vi "Stop.vi"(8 "error in (no error)":errorcluster, 9 "timeout in ms (-1)":i32=-1, 11 "Process In":refnum<class "Process.lvclass">) -> (0 "error out":errorcluster, 1 "timed out?":bool, 3 "Process Out":refnum<class "Process.lvclass">)   [LabVIEW 2020, in "Process.lvclass"]
doc: "Sends a stop message to the process, which must perform a safe shut down. This VI waits for the process to call the Finish method or times out if the configured time out expires."
uses:
  Process.lvclass
  Process.lvclass/Process.ctl
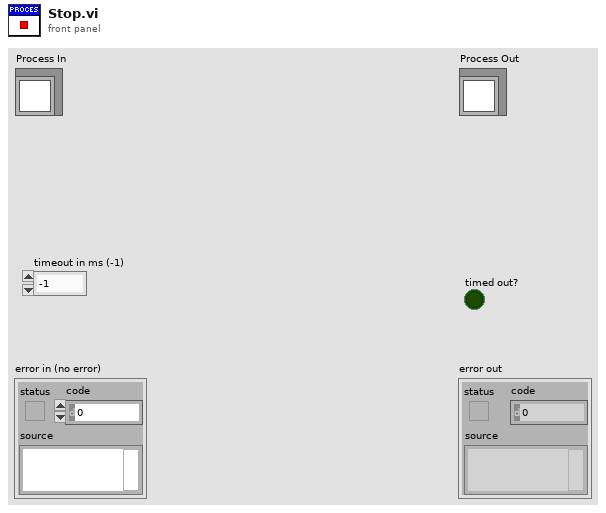
[diagram p1: front panel]
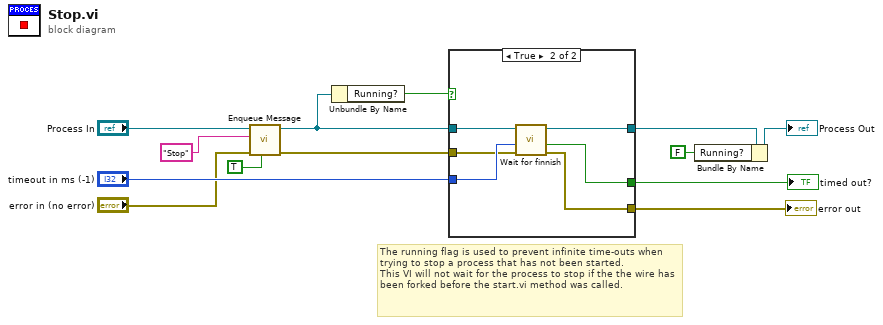
[diagram p0: block diagram]
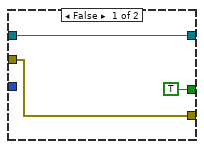
[diagram p2: hidden frame]
diagram:
  # "The running flag is used to prevent infinite time-outs when trying to stop a process that has not been started.\nThis VI will not wait for the process to stop if the the wire has been forked before the start.vi method was called."
  n1 = call "Enqueue Message.vi"("Priority Message? (F)"=TRUE, "error in (no error)"="error in (no error)", "Message"="Stop", "Process In"="Process In") -> ("error out"=w9:errorcluster, "Process Out"=w2:refnum<class "Process.lvclass">)  [unwired: 6 in]
  n2 = Unbundle By Name(w2) -> ("Running?"=w1:bool)
  n3 = case shown="True" w1 {
    tunnel: [w16 w22] -> w12
    tunnel: "timeout in ms (-1)" -> [_ w21]
    tunnel: [TRUE ("timed out?") w20] -> w10
    tunnel: w9 -> [w14 w19]
    tunnel: [w14 w18] -> w7
    tunnel: w2 -> [w16 w17]
    frame False {
    }
    frame True {
      n4 = call "Wait for finnish.vi"("error in (no error)"=w19, "timeout in ms (-1)"=w21, "Process In"=w17) -> ("error out"=w18:errorcluster, "timed out?"=w20:bool, "Process Out"=w22:refnum<class "Process.lvclass">)  [unwired: 6 in]
    }
  }
  "error out" <- w7
  "timed out?" <- w10
  n5 = Bundle By Name(cluster=w12, "Running?"=FALSE) -> (→"Process Out":refnum<class "Process.lvclass">)
